vi "Open VI by Path.vi"(6 "Block Diagram?":bool, 8 "error in":errorcluster, 10 "VI Path":path, 11 "Application in":refnum<vi>) -> (0 "error out":errorcluster)   [LabVIEW 2020, in "Panther Dashboard.lvlib"]
uses:
  Class/Library/Library.lvclass/Library.ctl
  Panther Dashboard.lvlib
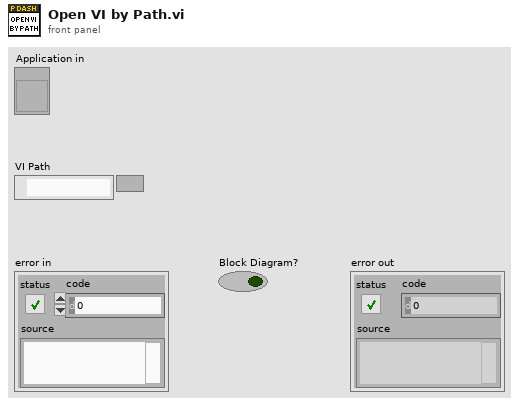
[diagram p1: front panel]
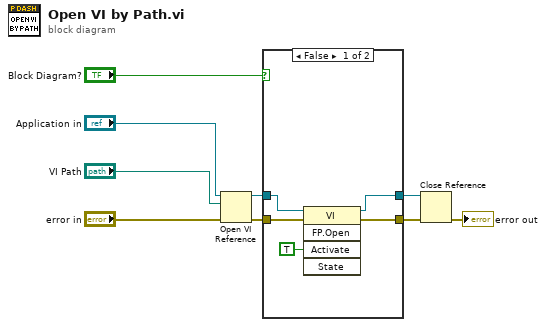
[diagram p0: block diagram]
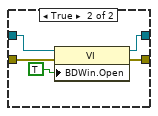
[diagram p2: hidden frame]
diagram:
  n1 = Open VI Reference(application reference (local)="Application in", vi path="VI Path", error in (no error)="error in") -> (vi reference=w2:refnum<vi>, error out=w7:errorcluster)  [unwired: 3 in]
  n2 = case shown="False" "Block Diagram?" {
    tunnel: [w11 w17] -> w3
    tunnel: w2 -> [w12 w16]
    tunnel: w7 -> [w14 w19]
    tunnel: [w13 w18] -> w6
    frame False {
      n3 = invoke class="VI" method="FP.Open"(reference=w12, error in=w14, "Activate"=TRUE ("Activate?")) -> (reference out=w11:refnum<vi>, error out=w13:errorcluster)  [unwired: 2 in, 3 out]
    }
    frame True {
      n4 = property on="Property Node" class="VI"(reference=w16, error in=w19, "BDWin.Open"=TRUE ("Block Diagram Window:Open")) -> (reference out=w17:refnum<vi>, error out=w18:errorcluster)
    }
  }
  n5 = Close Reference(reference=w3, error in (no error)=w6) -> (error out=→"error out":errorcluster)
